vi "Values_Hierarchy.vi"   [LabVIEW 2021]
uses:
  Abs_Types/Single Float/Abs_Single Float.lvclass
  Abs_Types/Double Float/Abs_Double Float.lvclass
  Abs_Types/Extended Float/Abs_Extended Float.lvclass
  Abs_Types/Complex Double Float/Abs_Complex Double Float.lvclass
  Abs_Types/Complex Extended Float/Abs_Complex Extended Float.lvclass
  Abs_Types/Complex Single Float/Abs_Complex Single Float.lvclass
  Abs_Types/I8 Integer/Abs_I8 Integer.lvclass
  Abs_Types/I16 Integer/Abs_I16 Integer.lvclass
  Abs_Types/I32 Integer/Abs_I32 Integer.lvclass
  Abs_Types/I64 Integer/Abs_I64 Integer.lvclass
  Abs_Types/U8 Integer/Abs_U8 Integer.lvclass
  Abs_Types/U16 Integer/Abs_U16 Integer.lvclass
  Abs_Types/U32 Integer/Abs_U32 Integer.lvclass
  Abs_Types/U64 Integer/Abs_U64 Integer.lvclass
  Abs_Types/Time/Abs_Time.lvclass
  Abs_Types/Boolean/Abs_Boolean.lvclass
  Abs_Types/String/Abs_String.lvclass
  Abs_Types/Variant/Abs_Variant.lvclass
  Abs_Types/Waveform/Abs_Waveform.lvclass
  Support/Bool/Const_Bool.lvclass
  Support/Str/Const_Str.lvclass
  Support/SGL/Const_SGL.lvclass
  Support/DBL/Const_DBL.lvclass
  Support/EXT/Const_EXT.lvclass
  Support/CPLX_SGL/Const_CPLX_SGL.lvclass
  Support/CPLX_DBL/Const_CPLX_DBL.lvclass
  Support/CPLX_EXT/Const_CPLX_EXT.lvclass
  Support/I8/Const_I8.lvclass
  Support/I16/Const_I16.lvclass
  Support/I32/Const_I32.lvclass
  Support/I64/Const_I64.lvclass
  Support/U8/Const_U8.lvclass
  Support/U16/Const_U16.lvclass
  Support/U32/Const_U32.lvclass
  Support/U64/Const_U64.lvclass
  Support/Time/Const_Time.lvclass
  Support/Curr_Time/Const_Current Time.lvclass
  Support/Variant/Const_Variant.lvclass
  Support/WFM/Const_WFM.lvclass
  Variables/Support/Bool/Var_Bool.lvclass
  Variables/Support/STR/Var_Str.lvclass
  Variables/Support/SGL/Var_SGL.lvclass
  Variables/Support/DBL/Var_DBL.lvclass
  Variables/Support/EXT/Var_EXT.lvclass
  Variables/Support/CPLX_SGL/Var_CPLX_SGL.lvclass
  Variables/Support/CPLX_DBL/Var_CPLX_DBL.lvclass
  Variables/Support/CPLX_EXT/Var_CPLX_EXT.lvclass
  Variables/Support/I8/Var_I8.lvclass
  Variables/Support/I16/Var_I16.lvclass
  Variables/Support/I32/Var_I32.lvclass
  Abs_Types/Boolean/Static Read.vi
  Abs_Types/Boolean/Static Write.vi
  Variables/Support/I64/Var_I64.lvclass
  Variables/Support/U8/Var_U8.lvclass
  Variables/Support/U16/Var_U16.lvclass
  Variables/Support/U32/Var_U32.lvclass
  Variables/Support/U64/Var_U64.lvclass
  Variables/Support/Time/Var_Time.lvclass
  Variables/Support/Variant/Var_Variant.lvclass
  Variables/Support/WFM/Var_WFM.lvclass
  Abs_Types/Double Float/Simple Read.vi
panel:
  # "SEE DIAGRAM\nFOR Hierarchy"
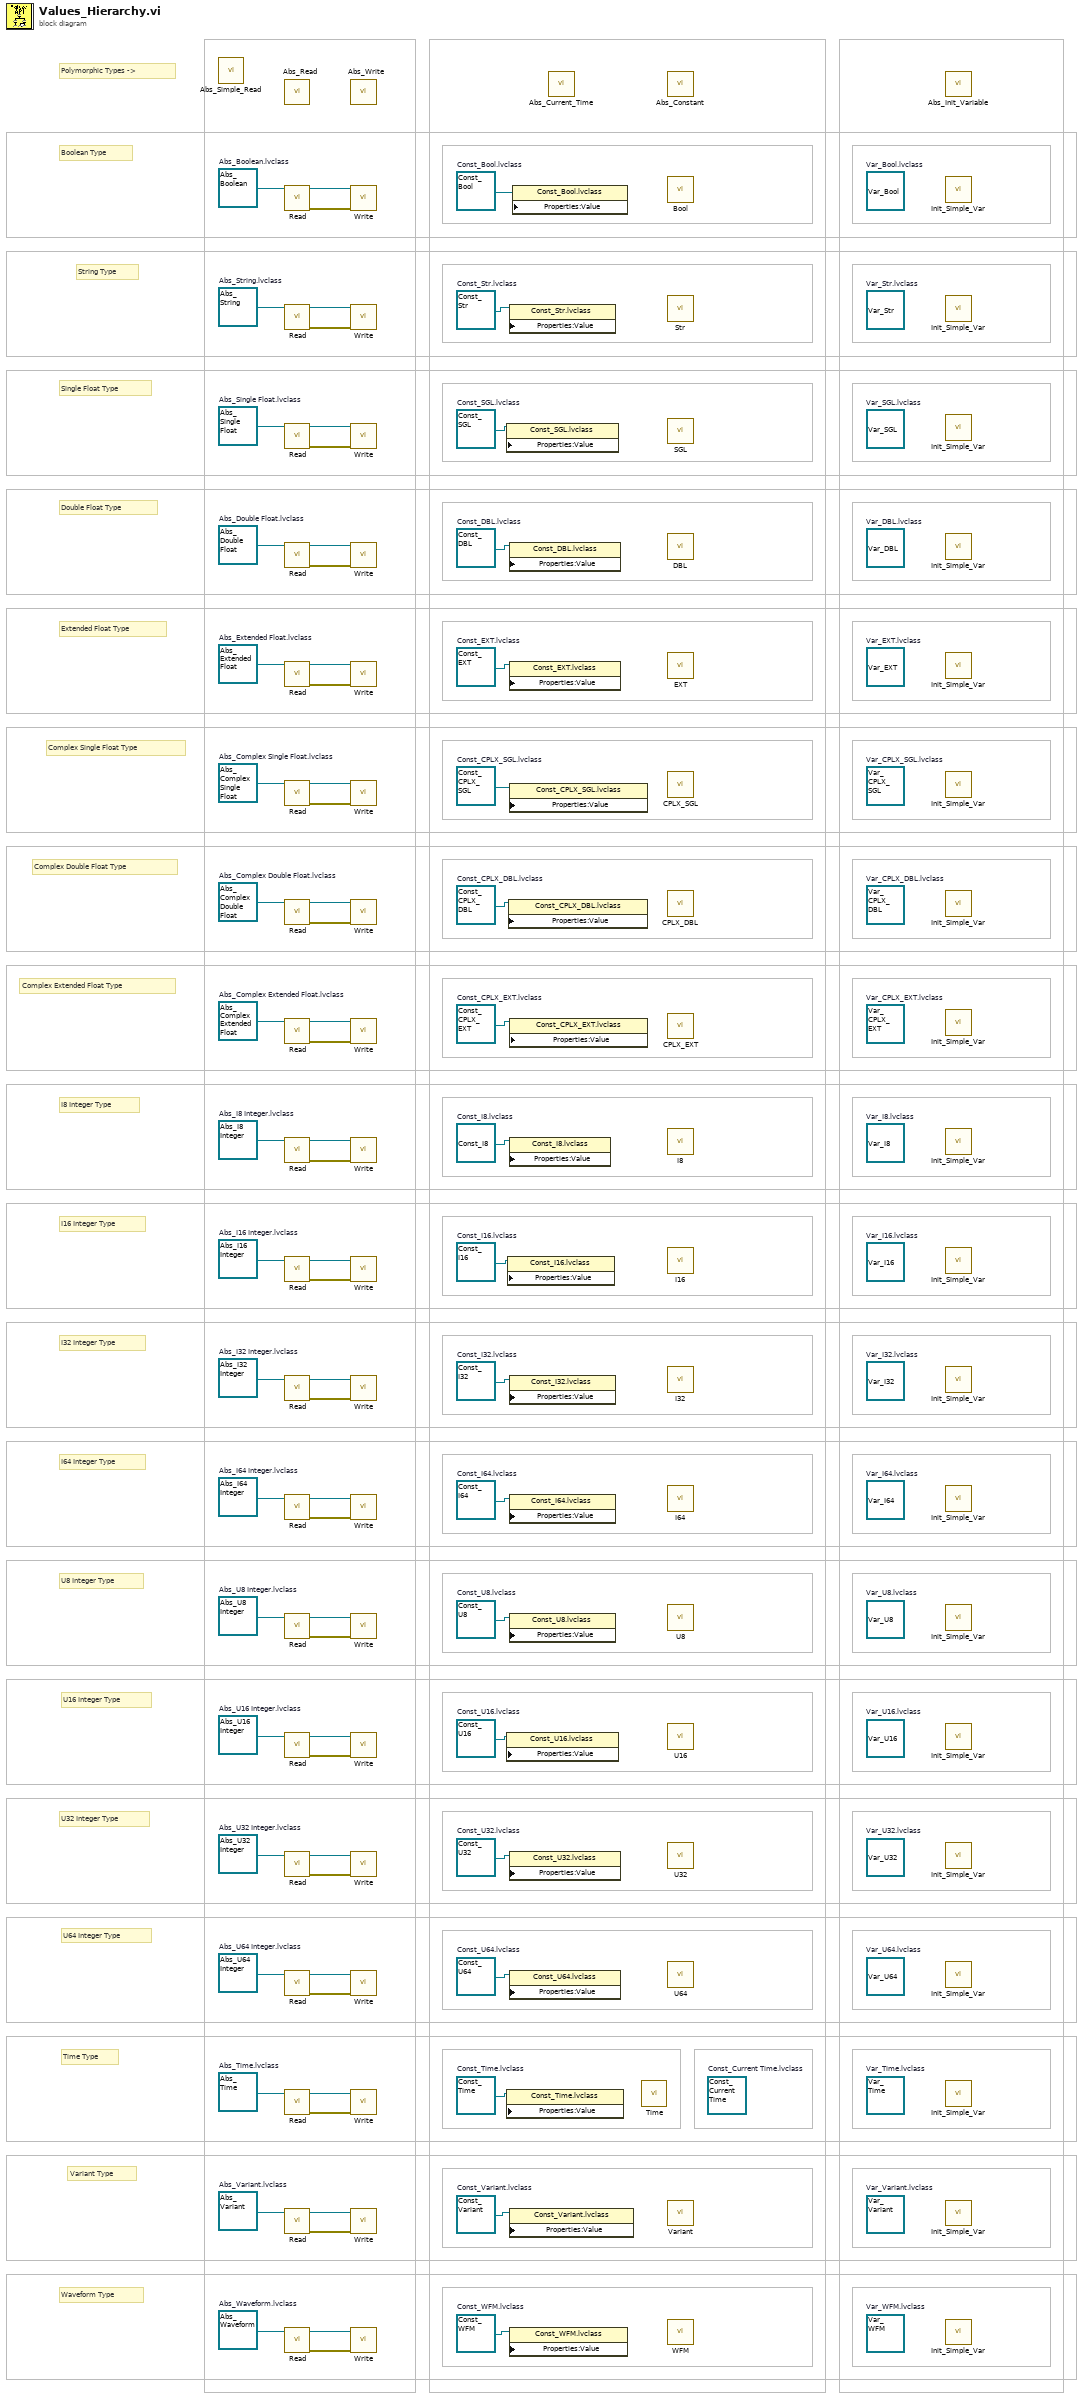
[diagram p0: block diagram]
diagram:
  (unwired) refnum<class "Var_WFM.lvclass"> refnum  # Var_WFM.lvclass
  (unwired) refnum<class "Var_Variant.lvclass"> refnum  # Var_Variant.lvclass
  (unwired) refnum<class "Var_Time.lvclass"> refnum  # Var_Time.lvclass
  (unwired) refnum<class "Var_U64.lvclass"> refnum  # Var_U64.lvclass
  (unwired) refnum<class "Var_U32.lvclass"> refnum  # Var_U32.lvclass
  (unwired) refnum<class "Var_U16.lvclass"> refnum  # Var_U16.lvclass
  (unwired) refnum<class "Var_U8.lvclass"> refnum  # Var_U8.lvclass
  (unwired) refnum<class "Var_I64.lvclass"> refnum  # Var_I64.lvclass
  (unwired) refnum<class "Var_I32.lvclass"> refnum  # Var_I32.lvclass
  (unwired) refnum<class "Var_I16.lvclass"> refnum  # Var_I16.lvclass
  (unwired) refnum<class "Var_I8.lvclass"> refnum  # Var_I8.lvclass
  (unwired) refnum<class "Var_CPLX_EXT.lvclass"> refnum  # Var_CPLX_EXT.lvclass
  (unwired) refnum<class "Var_CPLX_DBL.lvclass"> refnum  # Var_CPLX_DBL.lvclass
  (unwired) refnum<class "Var_CPLX_SGL.lvclass"> refnum  # Var_CPLX_SGL.lvclass
  (unwired) refnum<class "Var_EXT.lvclass"> refnum  # Var_EXT.lvclass
  (unwired) refnum<class "Var_DBL.lvclass"> refnum  # Var_DBL.lvclass
  (unwired) refnum<class "Var_SGL.lvclass"> refnum  # Var_SGL.lvclass
  (unwired) refnum<class "Var_Str.lvclass"> refnum  # Var_Str.lvclass
  (unwired) refnum<class "Var_Bool.lvclass"> refnum  # Var_Bool.lvclass
  w4 = refnum<class "Const_WFM.lvclass"> refnum  # Const_WFM.lvclass
  w5 = refnum<class "Const_Variant.lvclass"> refnum  # Const_Variant.lvclass
  (unwired) refnum<class "Const_Current Time.lvclass"> refnum  # Const_Current Time.lvclass
  w6 = refnum<class "Const_Time.lvclass"> refnum  # Const_Time.lvclass
  w7 = refnum<class "Const_U64.lvclass"> refnum  # Const_U64.lvclass
  w8 = refnum<class "Const_U32.lvclass"> refnum  # Const_U32.lvclass
  w9 = refnum<class "Const_U16.lvclass"> refnum  # Const_U16.lvclass
  w10 = refnum<class "Const_U8.lvclass"> refnum  # Const_U8.lvclass
  w11 = refnum<class "Const_I64.lvclass"> refnum  # Const_I64.lvclass
  w12 = refnum<class "Const_I32.lvclass"> refnum  # Const_I32.lvclass
  w13 = refnum<class "Const_I16.lvclass"> refnum  # Const_I16.lvclass
  w14 = refnum<class "Const_I8.lvclass"> refnum  # Const_I8.lvclass
  w15 = refnum<class "Const_CPLX_EXT.lvclass"> refnum  # Const_CPLX_EXT.lvclass
  w16 = refnum<class "Const_CPLX_DBL.lvclass"> refnum  # Const_CPLX_DBL.lvclass
  w17 = refnum<class "Const_CPLX_SGL.lvclass"> refnum  # Const_CPLX_SGL.lvclass
  w18 = refnum<class "Const_EXT.lvclass"> refnum  # Const_EXT.lvclass
  w19 = refnum<class "Const_DBL.lvclass"> refnum  # Const_DBL.lvclass
  w20 = refnum<class "Const_SGL.lvclass"> refnum  # Const_SGL.lvclass
  w21 = refnum<class "Const_Str.lvclass"> refnum  # Const_Str.lvclass
  w22 = refnum<class "Const_Bool.lvclass"> refnum  # Const_Bool.lvclass
  w30 = refnum<class "Abs_Waveform.lvclass"> refnum  # Abs_Waveform.lvclass
  w31 = refnum<class "Abs_Variant.lvclass"> refnum  # Abs_Variant.lvclass
  w36 = refnum<class "Abs_String.lvclass"> refnum  # Abs_String.lvclass
  w3 = refnum<class "Abs_Boolean.lvclass"> refnum  # Abs_Boolean.lvclass
  w23 = refnum<class "Abs_Time.lvclass"> refnum  # Abs_Time.lvclass
  w50 = refnum<class "Abs_U64 Integer.lvclass"> refnum  # Abs_U64 Integer.lvclass
  w49 = refnum<class "Abs_U32 Integer.lvclass"> refnum  # Abs_U32 Integer.lvclass
  w47 = refnum<class "Abs_U16 Integer.lvclass"> refnum  # Abs_U16 Integer.lvclass
  w48 = refnum<class "Abs_U8 Integer.lvclass"> refnum  # Abs_U8 Integer.lvclass
  w53 = refnum<class "Abs_I64 Integer.lvclass"> refnum  # Abs_I64 Integer.lvclass
  w52 = refnum<class "Abs_I32 Integer.lvclass"> refnum  # Abs_I32 Integer.lvclass
  w51 = refnum<class "Abs_I16 Integer.lvclass"> refnum  # Abs_I16 Integer.lvclass
  w58 = refnum<class "Abs_I8 Integer.lvclass"> refnum  # Abs_I8 Integer.lvclass
  w61 = refnum<class "Abs_Complex Single Float.lvclass"> refnum  # Abs_Complex Single Float.lvclass
  w64 = refnum<class "Abs_Complex Extended Float.lvclass"> refnum  # Abs_Complex Extended Float.lvclass
  w67 = refnum<class "Abs_Complex Double Float.lvclass"> refnum  # Abs_Complex Double Float.lvclass
  w70 = refnum<class "Abs_Extended Float.lvclass"> refnum  # Abs_Extended Float.lvclass
  w73 = refnum<class "Abs_Double Float.lvclass"> refnum  # Abs_Double Float.lvclass
  w76 = refnum<class "Abs_Single Float.lvclass"> refnum  # Abs_Single Float.lvclass
  # "Polymorphic Types ->"
  # "Waveform Type"
  # "Variant Type"
  # "Time Type"
  # "U64 Integer Type"
  # "U32 Integer Type"
  # "U16 Integer Type"
  # "U8 Integer Type"
  # "I64 Integer Type"
  # "I32 Integer Type"
  # "I16 Integer Type"
  # "I8 Integer Type"
  # "Complex Extended Float Type"
  # "Complex Double Float Type"
  # "Complex Single Float Type"
  # "Extended Float Type"
  # "Double Float Type"
  # "Single Float Type"
  # "String Type"
  # "Boolean Type"
  n1 = call-poly "Abs_Simple_Read.vi"() -> ()  [unwired: 5 in, 1 out]
  n2 = call-poly "Abs_Read.vi"() -> ()  [unwired: 9 in, 3 out]
  n3 = call-dynamic "Read.vi"("Boolean in"=w3) -> ("error out"=w37:errorcluster, "Boolean out"=w38:refnum<class "Abs_Boolean.lvclass">)  [unwired: 8 in, 1 out]
  n4 = call-dynamic "Read.vi"("Abs_String in"=w36) -> ("error out"=w34:errorcluster, "Abs_String out"=w35:refnum<class "Abs_String.lvclass">)  [unwired: 8 in, 1 out]
  n5 = call-dynamic "Read.vi"("Double Float.lvclass_340760 in"=w76) -> ("error out"=w74:errorcluster, "Double Float.lvclass_340760 out"=w75:refnum<class "Abs_Single Float.lvclass">)  [unwired: 8 in, 1 out]
  n6 = call-dynamic "Read.vi"("Double Float.lvclass_340760 in"=w73) -> ("error out"=w71:errorcluster, "Double Float.lvclass_340760 out"=w72:refnum<class "Abs_Double Float.lvclass">)  [unwired: 8 in, 1 out]
  n7 = call-dynamic "Read.vi"("Double Float.lvclass_340760 in"=w70) -> ("error out"=w68:errorcluster, "Double Float.lvclass_340760 out"=w69:refnum<class "Abs_Extended Float.lvclass">)  [unwired: 8 in, 1 out]
  n8 = call-dynamic "Read.vi"("Double Float.lvclass_340760 in"=w61) -> ("error out"=w59:errorcluster, "Double Float.lvclass_340760 out"=w60:refnum<class "Abs_Complex Single Float.lvclass">)  [unwired: 8 in, 1 out]
  n9 = call-dynamic "Read.vi"("Double Float.lvclass_340760 in"=w67) -> ("error out"=w65:errorcluster, "Double Float.lvclass_340760 out"=w66:refnum<class "Abs_Complex Double Float.lvclass">)  [unwired: 8 in, 1 out]
  n10 = call-dynamic "Read.vi"("Double Float.lvclass_340760 in"=w64) -> ("error out"=w62:errorcluster, "Double Float.lvclass_340760 out"=w63:refnum<class "Abs_Complex Extended Float.lvclass">)  [unwired: 8 in, 1 out]
  n11 = call-dynamic "Read.vi"("Double Float.lvclass_340760 in"=w58) -> ("error out"=w56:errorcluster, "Double Float.lvclass_340760 out"=w57:refnum<class "Abs_I8 Integer.lvclass">)  [unwired: 8 in, 1 out]
  n12 = call-dynamic "Read.vi"("Double Float.lvclass_340760 in"=w51) -> ("error out"=w25:errorcluster, "Double Float.lvclass_340760 out"=w27:refnum<class "Abs_I16 Integer.lvclass">)  [unwired: 8 in, 1 out]
  n13 = call-dynamic "Read.vi"("Double Float.lvclass_340760 in"=w52) -> ("error out"=w24:errorcluster, "Double Float.lvclass_340760 out"=w26:refnum<class "Abs_I32 Integer.lvclass">)  [unwired: 8 in, 1 out]
  n14 = call-dynamic "Read.vi"("Double Float.lvclass_340760 in"=w53) -> ("error out"=w54:errorcluster, "Double Float.lvclass_340760 out"=w55:refnum<class "Abs_I64 Integer.lvclass">)  [unwired: 8 in, 1 out]
  n15 = call-dynamic "Read.vi"("Double Float.lvclass_340760 in"=w48) -> ("error out"=w45:errorcluster, "Double Float.lvclass_340760 out"=w46:refnum<class "Abs_U8 Integer.lvclass">)  [unwired: 8 in, 1 out]
  n16 = call-dynamic "Read.vi"("Double Float.lvclass_340760 in"=w47) -> ("error out"=w43:errorcluster, "Double Float.lvclass_340760 out"=w44:refnum<class "Abs_U16 Integer.lvclass">)  [unwired: 8 in, 1 out]
  n17 = call-dynamic "Read.vi"("Double Float.lvclass_340760 in"=w49) -> ("error out"=w41:errorcluster, "Double Float.lvclass_340760 out"=w42:refnum<class "Abs_U32 Integer.lvclass">)  [unwired: 8 in, 1 out]
  n18 = call-dynamic "Read.vi"("Double Float.lvclass_340760 in"=w50) -> ("error out"=w1:errorcluster, "Double Float.lvclass_340760 out"=w2:refnum<class "Abs_U64 Integer.lvclass">)  [unwired: 8 in, 1 out]
  n19 = call-dynamic "Read.vi"("Double Float.lvclass_340760 in"=w23) -> ("error out"=w40:errorcluster, "Double Float.lvclass_340760 out"=w39:refnum<class "Abs_Time.lvclass">)  [unwired: 8 in, 1 out]
  n20 = call-dynamic "Read.vi"("Abs_Variant in"=w31) -> ("error out"=w32:errorcluster, "Abs_Variant out"=w33:refnum<class "Abs_Variant.lvclass">)  [unwired: 8 in, 1 out]
  n21 = call-dynamic "Read.vi"("Abs_Waveform in"=w30) -> ("error out"=w29:errorcluster, "Abs_Waveform out"=w28:refnum<class "Abs_Waveform.lvclass">)  [unwired: 8 in, 1 out]
  n22 = call-poly "Abs_Write.vi"() -> ()  [unwired: 10 in, 2 out]
  n23 = call-dynamic "Write.vi"("error in (no error)"=w37, "Boolean in"=w38) -> ()  [unwired: 8 in, 2 out]
  n24 = call-dynamic "Write.vi"("error in (no error)"=w34, "Abs_String in"=w35) -> ()  [unwired: 8 in, 2 out]
  n25 = call-dynamic "Write.vi"("error in (no error)"=w74, "Double Float.lvclass_340760 in"=w75) -> ()  [unwired: 8 in, 2 out]
  n26 = call-dynamic "Write.vi"("error in (no error)"=w71, "Double Float.lvclass in"=w72) -> ()  [unwired: 8 in, 2 out]
  n27 = call-dynamic "Write.vi"("error in (no error)"=w68, "Double Float.lvclass_340760 in"=w69) -> ()  [unwired: 8 in, 2 out]
  n28 = call-dynamic "Write.vi"("error in (no error)"=w59, "Double Float.lvclass_340760 in"=w60) -> ()  [unwired: 8 in, 2 out]
  n29 = call-dynamic "Write.vi"("error in (no error)"=w65, "Double Float.lvclass_340760 in"=w66) -> ()  [unwired: 8 in, 2 out]
  n30 = call-dynamic "Write.vi"("error in (no error)"=w62, "Double Float.lvclass_340760 in"=w63) -> ()  [unwired: 8 in, 2 out]
  n31 = call-dynamic "Write.vi"("error in (no error)"=w56, "Double Float.lvclass_340760 in"=w57) -> ()  [unwired: 8 in, 2 out]
  n32 = call-dynamic "Write.vi"("error in (no error)"=w25, "Double Float.lvclass_340760 in"=w27) -> ()  [unwired: 8 in, 2 out]
  n33 = call-dynamic "Write.vi"("error in (no error)"=w24, "Double Float.lvclass_340760 in"=w26) -> ()  [unwired: 8 in, 2 out]
  n34 = call-dynamic "Write.vi"("error in (no error)"=w54, "Double Float.lvclass_340760 in"=w55) -> ()  [unwired: 8 in, 2 out]
  n35 = call-dynamic "Write.vi"("error in (no error)"=w45, "Double Float.lvclass_340760 in"=w46) -> ()  [unwired: 8 in, 2 out]
  n36 = call-dynamic "Write.vi"("error in (no error)"=w43, "Double Float.lvclass_340760 in"=w44) -> ()  [unwired: 8 in, 2 out]
  n37 = call-dynamic "Write.vi"("error in (no error)"=w41, "Double Float.lvclass_340760 in"=w42) -> ()  [unwired: 8 in, 2 out]
  n38 = call-dynamic "Write.vi"("error in (no error)"=w1, "Double Float.lvclass_340760 in"=w2) -> ()  [unwired: 8 in, 2 out]
  n39 = call-dynamic "Write.vi"("error in (no error)"=w40, "Double Float.lvclass_340760 in"=w39) -> ()  [unwired: 8 in, 2 out]
  n40 = call-dynamic "Write.vi"("error in (no error)"=w32, "Abs_Variant in"=w33) -> ()  [unwired: 8 in, 2 out]
  n41 = call-dynamic "Write.vi"("error in (no error)"=w29, "Abs_Waveform in"=w28) -> ()  [unwired: 8 in, 2 out]
  n42 = property class="Const_SGL.lvclass" props=["Properties:Value"](reference=w20) -> ()  [unwired: 2 in, 2 out]
  n43 = property class="Const_U16.lvclass" props=["Properties:Value"](reference=w9) -> ()  [unwired: 2 in, 2 out]
  n44 = property class="Const_Time.lvclass" props=["Properties:Value"](reference=w6) -> ()  [unwired: 2 in, 2 out]
  n45 = property class="Const_I16.lvclass" props=["Properties:Value"](reference=w13) -> ()  [unwired: 2 in, 2 out]
  n46 = property class="Const_CPLX_DBL.lvclass" props=["Properties:Value"](reference=w16) -> ()  [unwired: 2 in, 2 out]
  n47 = property class="Const_Str.lvclass" props=["Properties:Value"](reference=w21) -> ()  [unwired: 2 in, 2 out]
  n48 = property class="Const_DBL.lvclass" props=["Properties:Value"](reference=w19) -> ()  [unwired: 2 in, 2 out]
  n49 = property class="Const_EXT.lvclass" props=["Properties:Value"](reference=w18) -> ()  [unwired: 2 in, 2 out]
  n50 = property class="Const_CPLX_SGL.lvclass" props=["Properties:Value"](reference=w17) -> ()  [unwired: 2 in, 2 out]
  n51 = property class="Const_I8.lvclass" props=["Properties:Value"](reference=w14) -> ()  [unwired: 2 in, 2 out]
  n52 = property class="Const_I32.lvclass" props=["Properties:Value"](reference=w12) -> ()  [unwired: 2 in, 2 out]
  n53 = property class="Const_I64.lvclass" props=["Properties:Value"](reference=w11) -> ()  [unwired: 2 in, 2 out]
  n54 = property class="Const_U8.lvclass" props=["Properties:Value"](reference=w10) -> ()  [unwired: 2 in, 2 out]
  n55 = property class="Const_U32.lvclass" props=["Properties:Value"](reference=w8) -> ()  [unwired: 2 in, 2 out]
  n56 = property class="Const_U64.lvclass" props=["Properties:Value"](reference=w7) -> ()  [unwired: 2 in, 2 out]
  n57 = property class="Const_Variant.lvclass" props=["Properties:Value"](reference=w5) -> ()  [unwired: 2 in, 2 out]
  n58 = property class="Const_WFM.lvclass" props=["Properties:Value"](reference=w4) -> ()  [unwired: 2 in, 2 out]
  n59 = property class="Const_CPLX_EXT.lvclass" props=["Properties:Value"](reference=w15) -> ()  [unwired: 2 in, 2 out]
  n60 = property class="Const_Bool.lvclass" props=["Properties:Value"](reference=w22) -> ()  [unwired: 2 in, 2 out]
  n61 = call "Abs_Current_Time.vi"() -> ()  [unwired: 5 in, 1 out]
  n62 = call "Time.vi"() -> ()  [unwired: 5 in, 1 out]
  n63 = call-poly "Abs_Constant.vi"() -> ()  [unwired: 5 in, 1 out]
  n64 = call "Bool.vi"() -> ()  [unwired: 5 in, 1 out]
  n65 = call "Str.vi"() -> ()  [unwired: 5 in, 1 out]
  n66 = call "SGL.vi"() -> ()  [unwired: 5 in, 1 out]
  n67 = call "DBL.vi"() -> ()  [unwired: 5 in, 1 out]
  n68 = call "EXT.vi"() -> ()  [unwired: 5 in, 1 out]
  n69 = call "CPLX_SGL.vi"() -> ()  [unwired: 5 in, 1 out]
  n70 = call "CPLX_DBL.vi"() -> ()  [unwired: 5 in, 1 out]
  n71 = call "CPLX_EXT.vi"() -> ()  [unwired: 5 in, 1 out]
  n72 = call "I8.vi"() -> ()  [unwired: 5 in, 1 out]
  n73 = call "I16.vi"() -> ()  [unwired: 5 in, 1 out]
  n74 = call "I32.vi"() -> ()  [unwired: 5 in, 1 out]
  n75 = call "I64.vi"() -> ()  [unwired: 5 in, 1 out]
  n76 = call "U8.vi"() -> ()  [unwired: 5 in, 1 out]
  n77 = call "U16.vi"() -> ()  [unwired: 5 in, 1 out]
  n78 = call "U32.vi"() -> ()  [unwired: 5 in, 1 out]
  n79 = call "U64.vi"() -> ()  [unwired: 5 in, 1 out]
  n80 = call "Variant.vi"() -> ()  [unwired: 5 in, 1 out]
  n81 = call "WFM.vi"() -> ()  [unwired: 5 in, 1 out]
  n82 = call-poly "Abs_Init_Variable.vi"() -> ()  [unwired: 5 in, 1 out]
  n83 = call "Init_Simple_Var.vi"() -> ()  [unwired: 5 in, 1 out]
  n84 = call "Init_Simple_Var.vi"() -> ()  [unwired: 5 in, 1 out]
  n85 = call "Init_Simple_Var.vi"() -> ()  [unwired: 5 in, 1 out]
  n86 = call "Init_Simple_Var.vi"() -> ()  [unwired: 5 in, 1 out]
  n87 = call "Init_Simple_Var.vi"() -> ()  [unwired: 5 in, 1 out]
  n88 = call "Init_Simple_Var.vi"() -> ()  [unwired: 5 in, 1 out]
  n89 = call "Init_Simple_Var.vi"() -> ()  [unwired: 5 in, 1 out]
  n90 = call "Init_Simple_Var.vi"() -> ()  [unwired: 5 in, 1 out]
  n91 = call "Init_Simple_Var.vi"() -> ()  [unwired: 5 in, 1 out]
  n92 = call "Init_Simple_Var.vi"() -> ()  [unwired: 5 in, 1 out]
  n93 = call "Init_Simple_Var.vi"() -> ()  [unwired: 5 in, 1 out]
  n94 = call "Init_Simple_Var.vi"() -> ()  [unwired: 5 in, 1 out]
  n95 = call "Init_Simple_Var.vi"() -> ()  [unwired: 5 in, 1 out]
  n96 = call "Init_Simple_Var.vi"() -> ()  [unwired: 5 in, 1 out]
  n97 = call "Init_Simple_Var.vi"() -> ()  [unwired: 5 in, 1 out]
  n98 = call "Init_Simple_Var.vi"() -> ()  [unwired: 5 in, 1 out]
  n99 = call "Init_Simple_Var.vi"() -> ()  [unwired: 5 in, 1 out]
  n100 = call "Init_Simple_Var.vi"() -> ()  [unwired: 5 in, 1 out]
  n101 = call "Init_Simple_Var.vi"() -> ()  [unwired: 5 in, 1 out]
